vi "Result Response.vi"(8 "error in (no error)":errorcluster, 10 "Acquired Result":refnum<class "Acquired Result.lvclass">, 11 "Measure Controller in":refnum<class "Process Controller.lvclass">) -> (0 "error out":errorcluster, 3 "Measure Controller out":refnum<class "Process Controller.lvclass">)   [LabVIEW 2016, in "Process Controller.lvclass"]
uses:
  Process Controller.lvclass
  C:/github/Measure_core/Template Module/Template Module.lvclass
  Results/Acquired Result/Acquired Result.lvclass
  Template Module/Template Module.lvclass/Template Module.ctl
  Template Module/Read tdms stream.vi
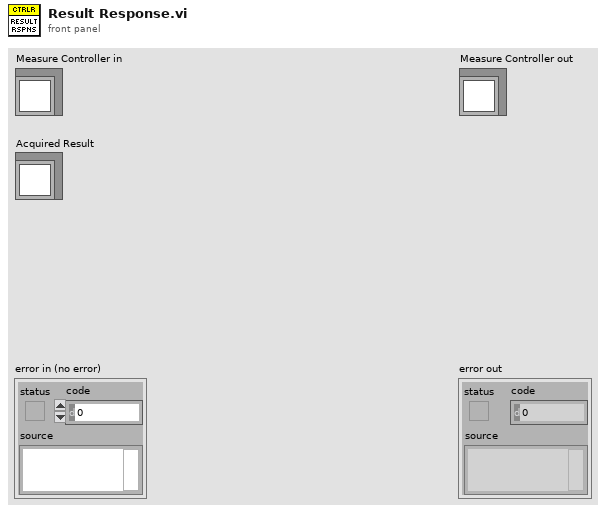
[diagram p1: front panel]
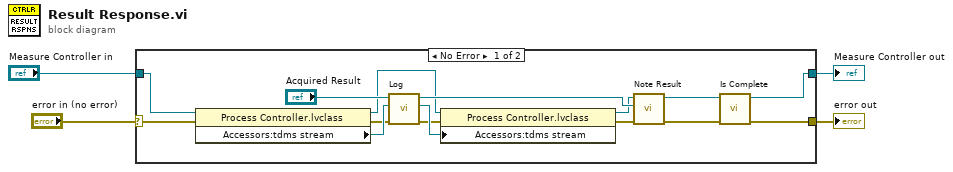
[diagram p0: block diagram]
diagram:
  n1 = case shown="No Error" "error in (no error)" {
    selector: "error in (no error)" -> [w10 w21]
    tunnel: [w18 w21] -> w3
    tunnel: [w19 w20] -> w1
    tunnel: "Measure Controller in" -> [w15 w20]
    frame No Error {
      n2 = property class="Process Controller.lvclass"(reference=w15, error in=w10) -> (reference out=w7:refnum<class "Process Controller.lvclass">, error out=w9:errorcluster, "Accessors:tdms stream"=w12:refnum<k34>)
      n3 = call-dynamic "Log.vi"("error in (no error)"=w9, "tdms file"=w12, "Acquired Result in"="Acquired Result") -> ("error out"=w8:errorcluster, "tdms file out"=w11:refnum<k34>, "Acquired Result out"=w13:refnum<class "Acquired Result.lvclass">)  [unwired: 6 in]
      n4 = property class="Process Controller.lvclass"(reference=w7, error in=w8, "Accessors:tdms stream"=w11) -> (reference out=w5:refnum<class "Process Controller.lvclass">, error out=w6:errorcluster)
      n5 = call-dynamic "Note Result.vi"("error in (no error)"=w6, "Acquired Result.lvclass"=w13, "Measure Controller in"=w5) -> ("error out"=w16:errorcluster, "Measure Controller out"=w17:refnum<class "Process Controller.lvclass">)  [unwired: 7 in]
      n6 = call-dynamic "Is Complete.vi"("error in (no error)"=w16, "Measure Controller in"=w17) -> ("error out"=w18:errorcluster, "Measure Controller out"=w19:refnum<class "Process Controller.lvclass">)  [unwired: 8 in]
    }
    frame Error {
    }
  }
  "error out" <- w3
  "Measure Controller out" <- w1
